vi "Double coinc 2 muon track.vi"(11 "Array of two hits":T1[](array[typedef])) -> (3 "Muon track":cluster{"Azimuth":dbl, "Polar":dbl})   [LabVIEW 2016]
uses:
  Typedefs/Coincidence.ctl
  <vilib>/Analysis/coordinate.llb/3D Coordinate Conversion (Scalar).vi
  <vilib>/Analysis/NI_AALPro.lvlib
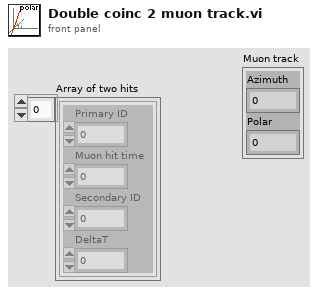
[diagram p1: front panel]
types:
  T1 = typedef "Coincidence.ctl" = cluster{"Primary ID":i8, "Muon hit time":u64, "Secondary ID":i8, "DeltaT":i32}
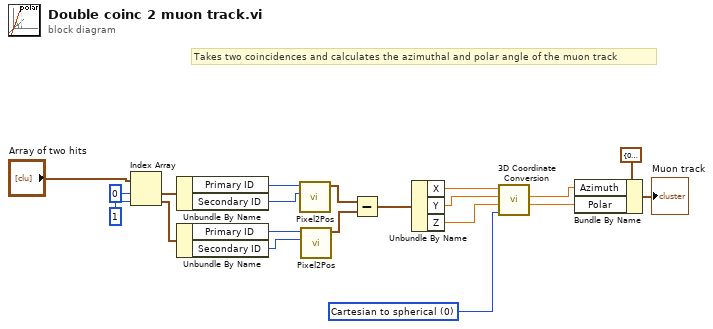
[diagram p0: block diagram]
diagram:
  w17 = u16 0 items=["Cartesian to spherical", "spherical to Cartesian", "Cartesian to cylindrical", "cylindrical to Cartesian", "spherical to cylindrical", "cylindrical to spherical"] ("conversion type")
  # "Takes two coincidences and calculates the azimuthal and polar angle of the muon track"
  n1 = Index Array(array="Array of two hits", index #1=0 ("index"), index #2=1 ("index")) -> (element #1=w4:T1, element #2=w6:T1)
  n2 = Unbundle By Name(w4) -> ("Primary ID"=w7:i8, "Secondary ID"=w8:i8)
  n3 = Unbundle By Name(w6) -> ("Primary ID"=w9:i8, "Secondary ID"=w10:i8)
  n4 = call "Pixel2Pos.vi"("Secondary"=w8, "Primary"=w7) -> ("Position (m)"=w14:cluster{"X":dbl, "\nY":dbl, "\nZ":dbl})  [unwired: 9 in]
  n5 = call "Pixel2Pos.vi"("Secondary"=w10, "Primary"=w9) -> ("Position (m)"=w15:cluster{"X":dbl, "\nY":dbl, "\nZ":dbl})  [unwired: 9 in]
  n6 = Subtract(x=w14, y=w15) -> (x-y=w16:cluster{"X":dbl, "\nY":dbl, "\nZ":dbl})
  n7 = Unbundle By Name(w16) -> ("X"=w11:dbl, "Y"=w12:dbl, "Z"=w13:dbl)
  n8 = call-poly <vilib>:"3D Coordinate Conversion.vi"("conversion type"=w17, "axis 3"=w13, "axis 2"=w12, "axis 1"=w11) -> ("axis 3 out"=w20:dbl, "axis 2 out"=w19:dbl)  [unwired: 4 in, 2 out]
  n9 = Bundle By Name(cluster=cluster{"Azimuth":dbl, "Polar":dbl} {"Azimuth"=0.0, "Polar"=0.0}, "Azimuth"=w19, "Polar"=w20) -> (→"Muon track":cluster{"Azimuth":dbl, "Polar":dbl})
